vi "I2C Playground LINXorMYRIO I2C bug - SOLUTION.vi"() -> ()   [LabVIEW 2014]
uses:
  <vilib>/myRIO/Instrument Drivers/Onboard IO/DIO/typedefs/DIO Reference.ctl
  <vilib>/myRIO/Common/Instrument Driver Framework/Utilities/typedefs/myRIO Generic Hardware Reference.ctl
  <vilib>/myRIO/Common/Instrument Driver Framework/Utilities/typedefs/Hardware Version Enum.ctl
  <vilib>/myRIO/Common/Instrument Driver Framework/Utilities/typedefs/myRIO v1.0 Reference.ctl
  <vilib>/myRIO/Common/Instrument Driver Framework/Utilities/typedefs/Generic FPGA Reference.ctl
  <vilib>/myRIO/Common/Instrument Driver Framework/myRIO v1.0/DIO/typedefs/DIO Channels List.ctl
  <vilib>/myRIO/Common/Instrument Driver Framework/myRIO v1.0/DIO/typedefs/DIO Channels Enum.ctl
  <vilib>/userdefined/High Color/nirio_resource_hc.ctl
  <vilib>/myRIO/Instrument Drivers/Onboard IO/I2C/typedefs/I2C User Configuration.ctl
  <vilib>/myRIO/Instrument Drivers/Onboard IO/I2C/typedefs/I2C Transfer Rate.ctl
  <vilib>/myRIO/Instrument Drivers/Onboard IO/I2C/typedefs/I2C Reference.ctl
  <vilib>/myRIO/Common/Instrument Driver Framework/myRIO v1.0/I2C/typedefs/I2C Channels Enum.ctl
  <vilib>/myRIO/Instrument Drivers/Onboard IO/I2C/typedefs/I2C Configuration.ctl
  Sensors/VL6180/VL6180X DEFS.ctl
  <vilib>/myRIO/Common/Instrument Driver Framework/Utilities/vis/Is FPGA Ref Available.vi
  <vilib>/myRIO/Common/Instrument Driver Framework/myRIO v1.0/DIO/vis/myRIO v1.1 Open DIO.vi
  <vilib>/myRIO/Instrument Drivers/Onboard IO/DIO/vis/Write.vi
  <vilib>/myRIO/Common/Instrument Driver Framework/myRIO v1.0/I2C/vis/myRIO v1.1 Open I2C.vi
  <vilib>/myRIO/Instrument Drivers/Onboard IO/I2C/vis/Configure.vi
  <vilib>/myRIO/Instrument Drivers/Onboard IO/I2C/vis/Write Read.vi
  <vilib>/myRIO/Common/Instrument Driver Framework/Utilities/vis/Validate Channels.vi
  <vilib>/myRIO/Common/Instrument Driver Framework/myRIO v1.0/DIO/vis/myRIO v1.0 Reserve DIO.vi
  <vilib>/MakerHub/LINX/Public/Utilities/Check Channel.vi
  <vilib>/myRIO/Common/Instrument Driver Framework/myRIO v1.0/I2C/vis/myRIO v1.0 Reserve I2C.vi
  <vilib>/myRIO/Common/Instrument Driver Framework/myRIO v1.0/Resource Manager/vis/myRIO v1.0 Reserve Channel List.vi
  <vilib>/myRIO/Common/Instrument Driver Framework/myRIO v1.0/DIO/vis/myRIO v1.0 Build MUX Configuration DIO.vi
  <vilib>/myRIO/Common/Instrument Driver Framework/myRIO v1.0/I2C/vis/myRIO v1.0 Build MUX Configuration I2C.vi
  <vilib>/myRIO/Common/Instrument Driver Framework/myRIO v1.0/Resource Manager/vis/myRIO v1.0 Reserve Channel.vi
  <vilib>/myRIO/Common/Instrument Driver Framework/myRIO v1.0/Resource Manager/vis/myRIO v1.0 Unreserve Channel.vi
  <vilib>/myRIO/Common/Instrument Driver Framework/myRIO v1.0/Resource Manager/vis/myRIO v1.0 Create Configuration List.vi
  <vilib>/myRIO/Common/Instrument Driver Framework/myRIO v1.0/Resource Manager/vis/myRIO v1.0 Build Mutex Name.vi
  <vilib>/Utility/VariantDataType/GetNumericInfo.vi
  <vilib>/Utility/error.llb/Error Cluster From Error Code.vi
  <vilib>/myRIO/Common/Instrument Driver Framework/myRIO v1.0/myRIO v1.1 Open.vi
  <vilib>/myRIO/Common/Instrument Driver Framework/Utilities/vis/IO Manager.vi
  <vilib>/myRIO/Common/Instrument Driver Framework/Utilities/vis/Configuration Manager.vi
  <vilib>/myRIO/Common/Instrument Driver Framework/myRIO v1.0/Resource Manager/vis/myRIO v1.0 Configure IO.vi
  <vilib>/myRIO/Common/Instrument Driver Framework/myRIO v1.0/myRIO v1.0 Close.vi
  <vilib>/myRIO/Common/Instrument Driver Framework/myRIO v1.0/DIO/vis/myRIO v1.0 Write DIO.vi
  <vilib>/MakerHub/LINX/Public/Utilities/Open Local.vi
  <vilib>/MakerHub/LINX/Private/Utilties/Generate Error.vi
  <vilib>/MakerHub/LINX/Private/Local IO/LinxI2cOpen.vi
  <vilib>/MakerHub/LINX/Private/Local IO/LinxI2cWrite.vi
  <vilib>/MakerHub/LINX/Private/Local IO/LinxI2cRead.vi
  <vilib>/myRIO/Common/Instrument Driver Framework/myRIO v1.0/I2C/vis/myRIO v1.0 Configure I2C.vi
  <vilib>/myRIO/Common/Instrument Driver Framework/myRIO v1.0/I2C/vis/myRIO v1.0 Write I2C.vi
  <vilib>/myRIO/Common/Instrument Driver Framework/myRIO v1.0/I2C/vis/myRIO v1.0 Read I2C.vi
  <vilib>/myRIO/Express VI/Onboard IO/DO/DO Express VI.xnode
  <vilib>/myRIO/Instrument Drivers/Onboard IO/DIO/vis/myRIO DIO Open.xnode
  <vilib>/myRIO/Express VI/Onboard IO/I2C/I2C Express VI.xnode
  <vilib>/myRIO/Instrument Drivers/Onboard IO/I2C/vis/myRIO I2C Open.xnode
  <vilib>/MakerHub/LINX/LMH-LINX.lvlib
  <vilib>/myRIO/Instrument Drivers/Onboard IO/DIO/DIO.lvlib
  <vilib>/myRIO/Instrument Drivers/Onboard IO/I2C/I2C.lvlib
panel:
  out "Ch1 Error":errorcluster
  out "Ch0 Error":errorcluster
  out "CH 1 Answer: supposed to be x78":u8 format="%02x"
  in  "Test Mode":T1(ring)=enum."LINX: Both CH0 & CH1"
  out "CH 0 Answer: supposed to be x01":u8 format="%02x"
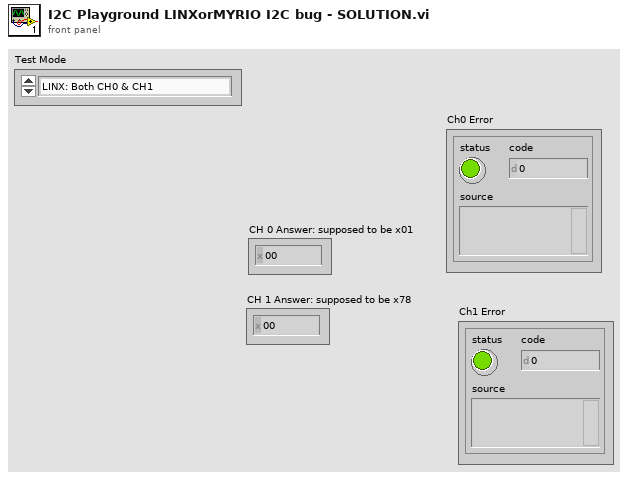
[diagram p1: front panel]
types:
  T1 = enum16{"Only CH 0", "Only CH 1", "LINX: Both CH0 & CH1", "myRIO ExpressVIs: Both "}
  T2 = typedef "LMH-LINX.lvlib/LINX Ref.ctl" = cluster{"IO":T3, "Interface":T4, "LINX Device Config":T5}
  T3 = typedef "LMH-LINX.lvlib/Platform.ctl" = enum16{"Remote", "Local"}
  T4 = typedef "LMH-LINX.lvlib/Interface.ctl" = enum16{"Serial", "TCP"}
  T5 = typedef "LMH-LINX.lvlib/Device.lvlib/LINX Device Config.ctl" = cluster{"Interface":T4, "COM Port":refnum<visa-resource-name>, "TCP Configuration":T6, "Device Family":u8, "Device ID":u8, "Device Name":string, "TCP Ref":refnum<k5>, "Channels":T7}
  T6 = typedef "LMH-LINX.lvlib/Device.lvlib/TCP Config.ctl" = cluster{"IP Address":string, "Port":u16}
  T7 = typedef "LMH-LINX.lvlib/Channels.ctl" = cluster{"DI":u8[], "DO":u8[], "AI":u8[], "AO":u8[], "PWM":u8[], "QE":u8[], "UART":u8[], "I2C 2":u8[], "SPI":u8[], "CAN":u8[], "Servo":u8[], "AI Ref (V)":dbl, "AI Resolution (Bits)":u8, "AO Ref (V)":dbl, "AO Resolution (Bits)":u8}
  T8 = typedef "I2C.lvlib/I2C Reference.ctl" = cluster{"myRIO Reference":T9, "I2C Channels Enum":T13, "I2C Configuration":T14}
  T9 = typedef "myRIO Generic Hardware Reference.ctl" = cluster{"myRIO Model":T10, "myRIO Hardware Reference":T11}
  T10 = typedef "Hardware Version Enum.ctl" = enum16{"Unknown", "myRIO-1900", "myRIO-1950"}
  T11 = typedef "myRIO v1.0 Reference.ctl" = cluster{"Generic FPGA Reference":T12, "Allow multiple opens":bool}
  T12 = typedef "Generic FPGA Reference.ctl" = refnum<k20>
  T13 = typedef "I2C Channels Enum.ctl" = enum16{"Not Connected", "A/I2C", "B/I2C"}
  T14 = typedef "I2C.lvlib/I2C Configuration.ctl" = cluster{"I2C Transfer Rate":T15}
  T15 = typedef "I2C.lvlib/I2C Transfer Rate.ctl" = enum16{"Standard mode (100 kbps)", "Fast mode (400 kbps)"}
  T16 = typedef "I2C.lvlib/I2C User Configuration.ctl" = cluster{"I2C Transfer Rate":T15}
  T17 = typedef "nirio_resource_hc.ctl" = tag
  T18 = typedef "VL6180X DEFS.ctl" = u16
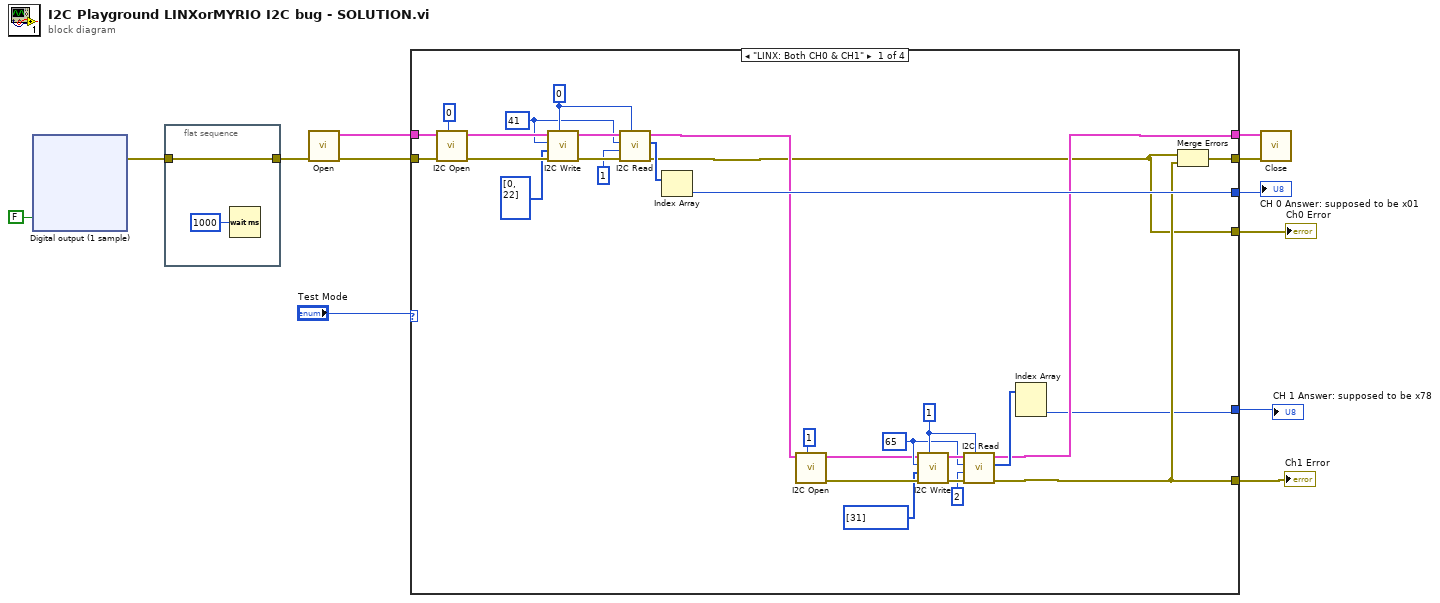
[diagram p0: block diagram]
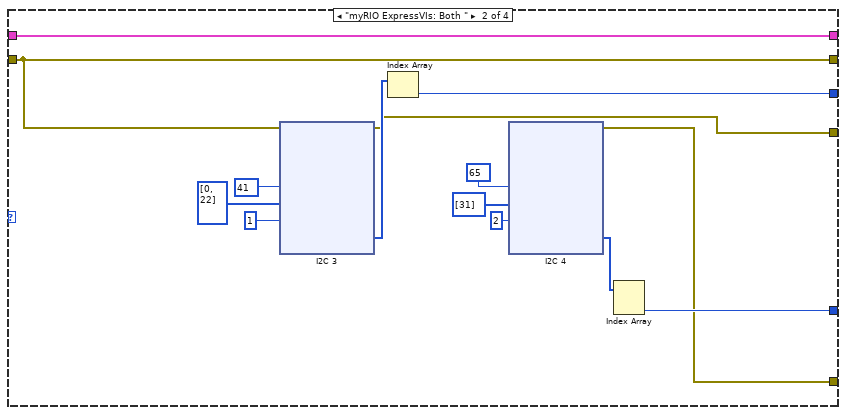
[diagram p2: hidden frame]
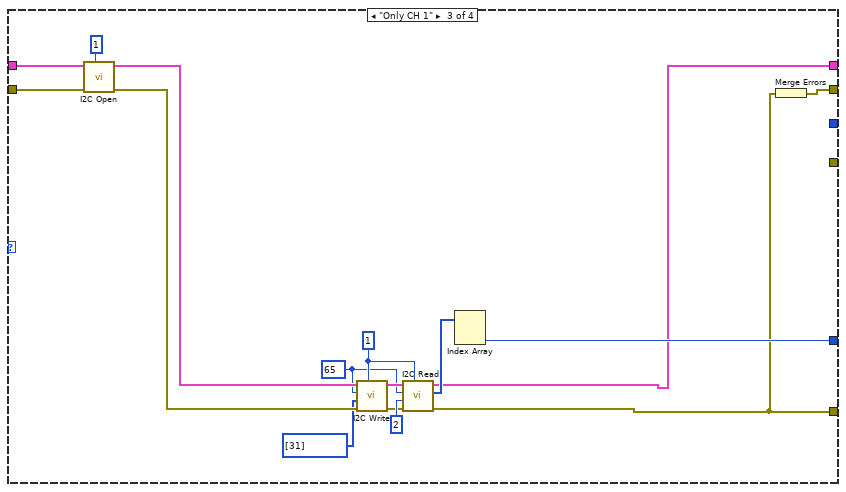
[diagram p3: hidden frame]
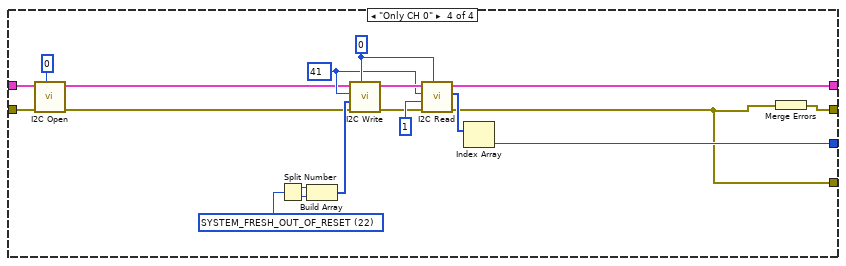
[diagram p4: hidden frame]
diagram:
  n1 = xnode "Digital output (1 sample)"("Sensor Power (B/DIO7 (Pin 25))"=FALSE) -> ("error out"=w2:errorcluster)  [unwired: 1 in]
  n2 = flat-sequence {
    tunnel: w2 -> [w13]
    tunnel: [w13] -> w1
    frame #0 {
      n3 = Wait (ms)(milliseconds to wait=u32 1000) -> ()  [unwired: 1 out]
    }
  }
  n4 = call-poly <vilib>:"Open.vi"("Error In"=w1) -> ("Error Out"=w12:errorcluster, "LINX Resource"=w11:T2)  [unwired: 8 in, 1 out]
  n5 = case shown="\"LINX: Both CH0 & CH1\"" "Test Mode" {
    tunnel: w12 -> [w39 w46 w140 w171]
    tunnel: w11 -> [w40 w47 w141 w170]
    tunnel: [w19 w47 w139 w155] -> w10
    tunnel: [w41 w46 w143 w159] -> w9
    tunnel: [w16 w45 _ w154] -> w6
    tunnel: [w18 w44 w138 _] -> w5
    tunnel: [w15 w56 w142 _] -> w4
    tunnel: [w21 w57 _ w158] -> w3
    frame "LINX: Both CH0 & CH1" {
      w25 = u8 65 ("I2C Slave Address (0)")
      w28 = u8 1 ("I2C Channel (0)")
      w32 = u8 41 ("I2C Slave Address (0)")
      w33 = u8 0 ("I2C Channel (0)")
      n6 = call <vilib>:"I2C Open.vi"("I2C Channel (0)"=u8 0, "Error In"=w39, "LINX Resource"=w40) -> ("Error Out"=w38:errorcluster, "LINX Resource"=w36:T2)  [unwired: 7 in]
      n7 = call <vilib>:"I2C Write.vi"("I2C Channel"=w33, "Error In"=w38, "Data"=u8[] [0, 22] ("appended array"), "I2C Slave Address (0)"=w32, "LINX Resource"=w36) -> ("Error Out"=w35:errorcluster, "LINX Resource"=w34:T2)  [unwired: 5 in]
      n8 = call <vilib>:"I2C Read.vi"("I2C Channel"=w33, "Error In"=w35, "Bytes To Read"=u8 1, "I2C Slave Address (0)"=w32, "LINX Resource"=w34) -> ("Error Out"=w16:errorcluster, "Data"=w29:u8[], "LINX Resource"=w17:T2)  [unwired: 4 in]
      n9 = Index Array(array=w29) -> (element=w21:u8)  [unwired: 1 in]
      n10 = call <vilib>:"I2C Open.vi"("I2C Channel (0)"=u8 1, "LINX Resource"=w17) -> ("Error Out"=w37:errorcluster, "LINX Resource"=w20:T2)  [unwired: 8 in]
      n11 = call <vilib>:"I2C Write.vi"("I2C Channel"=w28, "Error In"=w37, "Data"=u8[] [31], "I2C Slave Address (0)"=w25, "LINX Resource"=w20) -> ("Error Out"=w26:errorcluster, "LINX Resource"=w27:T2)  [unwired: 5 in]
      n12 = call <vilib>:"I2C Read.vi"("I2C Channel"=w28, "Error In"=w26, "Bytes To Read"=u8 2, "I2C Slave Address (0)"=w25, "LINX Resource"=w27) -> ("Error Out"=w18:errorcluster, "Data"=w22:u8[], "LINX Resource"=w19:T2)  [unwired: 4 in]
      n13 = Index Array(array=w22) -> (element #2=w15:u8)  [unwired: 2 in, 1 out]
      n14 = Merge Errors(w16, w18) -> (w41:errorcluster)
    }
    frame "myRIO ExpressVIs: Both " {
      n15 = xnode "I2C 3"("Slave Address (7-bit)"=u8 41 ("I2C Slave Address (0)"), "Bytes to Write"=u8[] [0, 22] ("appended array"), "Byte Count"=u8 1 ("Bytes To Read"), "error in (no error)"=w46) -> ("Bytes Read"=w53:u8[], "error out"=w45:errorcluster)
      n16 = Index Array(array=w53) -> (element=w57:u8)  [unwired: 1 in]
      n17 = xnode "I2C 4"("Slave Address (7-bit)"=u8 65 ("I2C Slave Address (0)"), "Bytes to Write"=u8[] [31] ("Data"), "Byte Count"=u8 2 ("Bytes To Read")) -> ("Bytes Read"=w48:u8[], "error out"=w44:errorcluster)  [unwired: 1 in]
      n18 = Index Array(array=w48) -> (element #2=w56:u8)  [unwired: 2 in, 1 out]
    }
    frame "Only CH 1" {
      w145 = u8 65 ("I2C Slave Address (0)")
      w146 = u8 1 ("I2C Channel (0)")
      n19 = call <vilib>:"I2C Open.vi"("I2C Channel (0)"=u8 1, "Error In"=w140, "LINX Resource"=w141) -> ("Error Out"=w147:errorcluster, "LINX Resource"=w148:T2)  [unwired: 7 in]
      n20 = call <vilib>:"I2C Write.vi"("I2C Channel"=w146, "Error In"=w147, "Data"=u8[] [31], "I2C Slave Address (0)"=w145, "LINX Resource"=w148) -> ("Error Out"=w152:errorcluster, "LINX Resource"=w151:T2)  [unwired: 5 in]
      n21 = call <vilib>:"I2C Read.vi"("I2C Channel"=w146, "Error In"=w152, "Bytes To Read"=u8 2, "I2C Slave Address (0)"=w145, "LINX Resource"=w151) -> ("Error Out"=w138:errorcluster, "Data"=w150:u8[], "LINX Resource"=w139:T2)  [unwired: 4 in]
      n22 = Index Array(array=w150) -> (element #2=w142:u8)  [unwired: 2 in, 1 out]
      n23 = Merge Errors(w138) -> (w143:errorcluster)
    }
    frame "Only CH 0" {
      w160 = u8 41 ("I2C Slave Address (0)")
      w161 = u8 0 ("I2C Channel (0)")
      w163 = T18 22 items=["IDENTIFICATION_MODEL_ID"=0, "IDENTIFICATION_MODEL_REV_MAJOR"=1, "IDENTIFICATION_MODEL_REV_MINOR"=2, "IDENTIFICATION_MODULE_REV_MAJOR"=3, "IDENTIFICATION_MODULE_REV_MINOR"=4, "IDENTIFICATION_DATE"=6, "IDENTIFICATION_TIME"=8, "SYSTEM_MODE_GPIO0"=16, "SYSTEM_MODE_GPIO1"=17, "SYSTEM_HISTORY_CTRL"=18, "SYSTEM_INTERRUPT_CONFIG_GPIO"=20, "SYSTEM_INTERRUPT_CLEAR"=21, "SYSTEM_FRESH_OUT_OF_RESET"=22, "SYSTEM_GROUPED_PARAMETER_HOLD"=23, "SYSRANGE_START"=24, "SYSRANGE_THRESH_HIGH"=25, "SYSRANGE_THRESH_LOW"=26, "SYSRANGE_INTERMEASUREMENT_PERIOD"=27, "SYSRANGE_MAX_CONVERGENCE_TIME"=28, "SYSRANGE_CROSSTALK_COMPENSATION_RATE"=30, "SYSRANGE_CROSSTALK_VALID_HEIGHT"=33, "SYSRANGE_EARLY_CONVERGENCE_ESTIMATE"=34, "SYSRANGE_PART_TO_PART_RANGE_OFFSET"=36, "SYSRANGE_RANGE_IGNORE_VALID_HEIGHT"=37, "SYSRANGE_RANGE_IGNORE_THRESHOLD"=38, "SYSRANGE_MAX_AMBIENT_LEVEL_MULT"=44, "SYSRANGE_RANGE_CHECK_ENABLES"=45, "SYSRANGE_VHV_RECALIBRATE"=46, "SYSRANGE_VHV_REPEAT_RATE"=49, "SYSALS_START"=56, "SYSALS_THRESH_HIGH"=58, "SYSALS_THRESH_LOW"=60, "SYSALS_INTERMEASUREMENT_PERIOD"=62, "SYSALS_ANALOGUE_GAIN"=63, "SYSALS_INTEGRATION_PERIOD"=64, "RESULT_RANGE_STATUS"=77, "RESULT_ALS_STATUS"=78, "RESULT_INTERRUPT_STATUS_GPIO"=79, "RESULT_ALS_VAL"=80, "RESULT_HISTORY_BUFFER"=82, "RESULT_RANGE_VAL"=98, "RESULT_RANGE_RAW"=100, "RESULT_RANGE_RETURN_RATE"=102, "RESULT_RANGE_REFERENCE_RATE"=104, "RESULT_RANGE_RETURN_SIGNAL_COUNT"=108, "RESULT_RANGE_REFERENCE_SIGNAL_COUNT"=112, "RESULT_RANGE_RETURN_AMB_COUNT"=116, "RESULT_RANGE_REFERENCE_AMB_COUNT"=120, "RESULT_RANGE_RETURN_CONV_TIME"=124, "RESULT_RANGE_REFERENCE_CONV_TIME"=128, "READOUT_AVERAGING_SAMPLE_PERIOD"=266, "FIRMWARE_BOOTUP"=281, "FIRMWARE_RESULT_SCALER"=288, "I2C_SLAVE_DEVICE_ADDRESS"=530, "INTERLEAVED_MODE_ENABLE"=675] ("VL6180X Constants")
      n24 = call <vilib>:"I2C Open.vi"("I2C Channel (0)"=u8 0, "Error In"=w171, "LINX Resource"=w170) -> ("Error Out"=w156:errorcluster, "LINX Resource"=w157:T2)  [unwired: 7 in]
      n25 = Split Number(x=w163) -> (hi(x)=w167:u8, lo(x)=w168:u8)
      n26 = Build Array(w167, w168) -> (w169:u8[])
      n27 = call <vilib>:"I2C Write.vi"("I2C Channel"=w161, "Error In"=w156, "Data"=w169, "I2C Slave Address (0)"=w160, "LINX Resource"=w157) -> ("Error Out"=w164:errorcluster, "LINX Resource"=w162:T2)  [unwired: 5 in]
      n28 = call <vilib>:"I2C Read.vi"("I2C Channel"=w161, "Error In"=w164, "Bytes To Read"=u8 1, "I2C Slave Address (0)"=w160, "LINX Resource"=w162) -> ("Error Out"=w154:errorcluster, "Data"=w166:u8[], "LINX Resource"=w155:T2)  [unwired: 4 in]
      n29 = Index Array(array=w166) -> (element=w158:u8)  [unwired: 1 in]
      n30 = Merge Errors(w154) -> (w159:errorcluster)
    }
  }
  "Ch0 Error" <- w6
  "Ch1 Error" <- w5
  "CH 1 Answer: supposed to be x78" <- w4
  "CH 0 Answer: supposed to be x01" <- w3
  n31 = call <vilib>:"Close.vi"("Error In"=w9, "LINX Resource"=w10) -> ()  [unwired: 9 in, 1 out]
